vi "dump.vi"(8 "error in (no error)":errorcluster, 10 "indent":T1, 11 "OpaqueDialectType in":refnum<class "OpaqueDialectType.lvclass">) -> (0 "error out":errorcluster, 2 "mlir":string, 3 "OpaqueDialectType out":refnum<class "OpaqueDialectType.lvclass">)   [LabVIEW 2020, in "mlir.lvlib" / "OpaqueDialectType.lvclass"]
uses:
  OpaqueDialectType.lvclass
  Node/indent.ctl
  OpaqueDialectType.lvclass/OpaqueDialectType.ctl
  mlir.lvlib
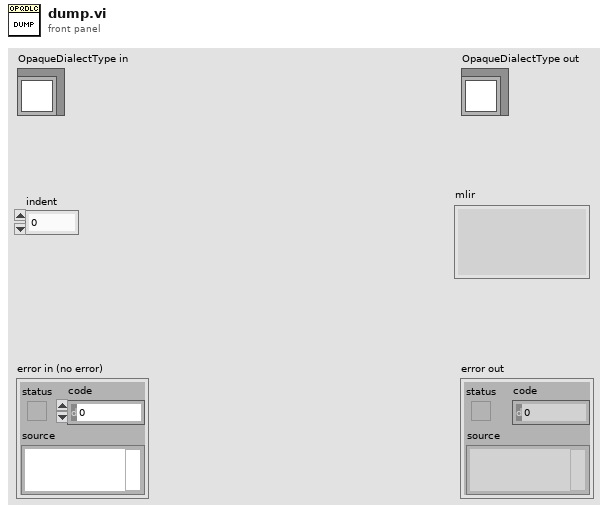
[diagram p1: front panel]
types:
  T1 = typedef "mlir.lvlib/indent.ctl" = u32
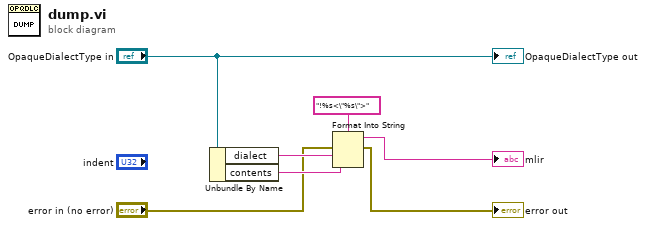
[diagram p0: block diagram]
diagram:
  n1 = Unbundle By Name("OpaqueDialectType in") -> ("dialect"=w7:string, "contents"=w6:string)
  n2 = Format Into String(format string="!%s<\"%s\">", error in="error in (no error)", w7, w6) -> (resulting string=→"mlir":string, error out=→"error out":errorcluster)  [unwired: 1 in]
  "OpaqueDialectType out" <- "OpaqueDialectType in"
